vi "Dashboard Main.vi"() -> ()   [LabVIEW 2019]
uses:
  <vilib>/Utility/miscctls.llb/LVRowAndColumnTypeDef.ctl
  <vilib>/event_ctls.llb/eventvkey.ctl
  <vilib>/Rock Robotics/Network Tables/NT Read Numeric Array.vi
  <vilib>/Rock Robotics/WPI/Dashboard/WPI_DashboardLogging Global.vi
  <vilib>/Rock Robotics/Network Tables/NT Write Boolean.vi
panel:
  in  "Camera Settings Right":T1={"Frame Rate"=30, "Compression"=30, "Size"=1, "DB Camera Config"=FALSE} {"Frame Rate" scale=1.0..30.0; "Compression" scale=100.0..-1.0; "Size" items=["640x480", "320x240", "160x120"]}
  in  "Camera Name Right":string(combo)="No Camera Selection"
  out "Camera Perf":string
  in  "Camera Settings":T1={"Frame Rate"=30, "Compression"=30, "Size"=1, "DB Camera Config"=FALSE} {"Frame Rate" scale=1.0..30.0; "Compression" scale=100.0..-1.0; "Size" items=["640x480", "320x240", "160x120"]}
  in  "TCP":refnum<k5>
  in  "Rec Mode":enum32{"Stop", "Record", "Playback"}(radio)
  out "Robot IP":string
  out "Image Message":string="Timeout in Camera Communications"
  in  "Dashboard Tab":T2(tab)
  in  "Enable Vision":bool=TRUE
  out "Vision Enabled":bool=TRUE
  in  "Select Auto":string(combo)="Select Autonomous ..."
  out "NT Connection":bool
  out "MotorChart R":cluster{"Numeric":dbl, "Numeric":dbl}(graph)
  out "MotorChart L":cluster{"Numeric":dbl, "Numeric":dbl}(graph)
  out "MotorSliders R":cluster{"MotorSlide1":dbl, "MotorSlide2":dbl} {"MotorSlide2" scale=-1.0..1.0 scale format="%#_2e"; "MotorSlide1" scale=-1.0..1.0 scale format="%#_2e"}
  out "MotorSliders L":cluster{"MotorSlide1":dbl, "MotorSlide2":dbl} {"MotorSlide2" scale=-1.0..1.0 scale format="%#_2e"; "MotorSlide1" scale=-1.0..1.0 scale format="%#_2e"}
  out "JS1 Z":dbl(slide) scale=-1.0..1.0 scale format="%#_2e"
  out "JS1 Graph":cluster{"X":dbl, "Y":dbl}[](graph)
  out "JS1 Buttons":T3
  out "JS2 Z":dbl(slide) scale=-1.0..1.0 scale format="%#_2e"
  out "JS2 Graph":cluster{"X":dbl, "Y":dbl}[](graph)
  out "JS2 Buttons":T3
  out "Mode":T4(ring)=enum."Auto Disabled"
  out "Right Camera Perf":cluster{"Bandwidth (Mbps)":dbl, "FPS":dbl}
  out "Top RPM":dbl caption="DB/String 1"
  out "Bottom RPM":dbl caption="DB/String 1"
  out "Camera Image Right":T5(plugin-control)
  out "Target Distance":dbl
  out "Skew":dbl caption="DB/String 1"
  out "Area":dbl caption="DB/String 1"
  out "Offset X":dbl
  out "Offset Y":dbl
  in  "Test Slider":dbl(slide) scale=0.0..100.0 scale format="%#_3g"
  in  "On/Off":bool caption="Solenoid"
  in  "Test Name":u16(ring) items=["Select the test to run..."]
  in  "Test Tree":string(tree)
  in  "Motor":cluster{"Value":dbl, "Enable":bool} {"Value" scale=-1.0..1.0 scale format="%#_3g"}
  out "Progress":T6 {"Test Progress" scale=0.0..100.0}
  in  "Rev/Fwd":cluster{"Forward":bool, "Reverse":bool}
  in  "Test Ring":u16(ring) items=["Monochrome", "Color"]
  out "Cmd Status":string
  in  "Execute Command":bool
  in  "Command Params":string[][](table)
  in  "Command Selection":i32(listbox)
  in  "CheckList":i32(listbox)
  out "Tree":string(tree)
  out "Camera Image":T5(plugin-control)
  out "Background":bool
  in  "Camera Name":string(combo)="No Camera Selection"
  # "HW"
  # "HW"
  # "Operator 1"
  # "Operator 2"
  # "Drive Motors"
  # "Front"
  # "Right"
  # "Left"
  # "Back"
  # "This tab is a great place for autonomous settings and robot-specific values.\nPlace controls and indicators inside this tab and match name to\nDashboard Variables on robot. You can also delete this comment."
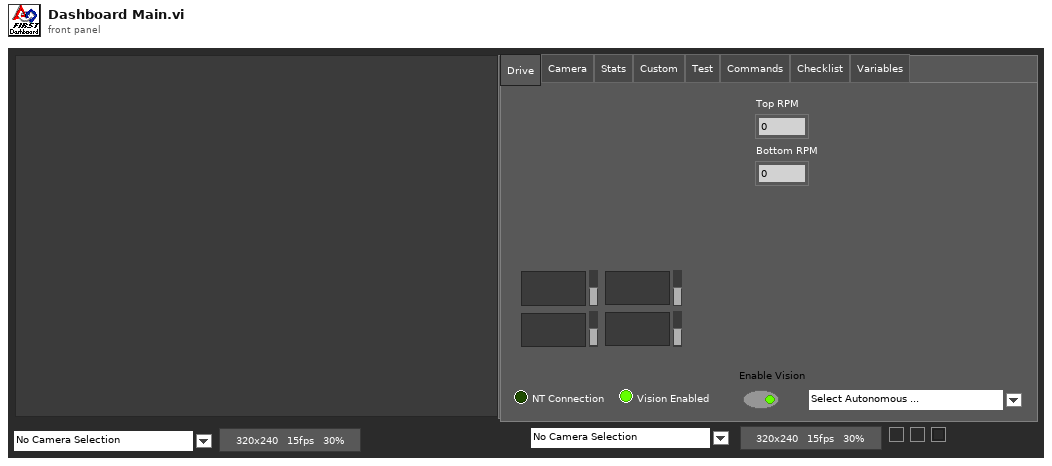
[diagram p1: front panel]
types:
  T1 = cluster{"Frame Rate":i32, "Compression":i32, "Size":u16, "DB Camera Config":bool}
  T2 = enum32{"Drive", "Camera", "Stats", "Custom", "Test", "Commands", "Checklist", "Variables"}
  T3 = cluster{bool, bool, bool, bool, bool, bool, bool, bool, bool, bool, bool, bool}
  T4 = enum8{"Tele-Op Disabled", "Tele-Op Enabled", "Auto Disabled", "Auto Enabled", "Test Disabled", "Test Enabled", "Disconnected", "No Code", "E-Stop"}
  T5 = typedef "IMAQ Image.ctl" = refnum<image>
  T6 = cluster{"Test Progress":u8, "Test Progress Text":string}
  T7 = cluster{"Save Path":path, "Interval (s)":dbl, "Keep":i32}
  T8 = enum32{"Drive", "Camera", "Basic", "Custom", "Test", "Commands", "Checklist", "Variables"}
  T9 = typedef "Image Type" = u32
  T10 = cluster{"IDs":cluster{"RPC field ID":u16, "Unique ID":u16}, "String":string}
  T11 = cluster{"Camera Image":refnum<vi>, "Dashboard Tab":refnum<vi>, "Background":refnum<vi>, "Rec Mode":refnum<vi>, "Test Slider":refnum<vi>, "On/Off ":refnum<vi>, "Test Ring":refnum<vi>, "Rev/Fwd":refnum<vi>, "Test Name":refnum<vi>, "Motor":refnum<vi>, "Progress":refnum<vi>, "CheckList":refnum<vi>, "Tree":refnum<vi>, "Test Tree":refnum<vi>, "Command Params":refnum<vi>, "Command Selection":refnum<vi>, "Execute Command":refnum<vi>, "Cmd Status":refnum<vi>, "Camera Settings":refnum<vi>, "Camera Name":refnum<vi>, "Camera Perf":refnum<vi>, "Camera Settings Right":refnum<vi>, "Camera Name Right":refnum<vi>, "Camera Image Right":refnum<vi>}
  T12 = cluster{"Global Rectangle":i32[], "Contours":cluster{"Contour Type":u32, "ROI Type":u32, "Points":i32[]}[]}
  T13 = cluster{"Camera Name Right":string, string, "Saved DB Images Info":cluster{"Save Path":path, "Interval (s)":dbl, "Keep":i32}}
  T14 = cluster{"Error Strings":string, "Disable Counts":cluster{u16, u16}, "Rail Faults":cluster{u16, u16, u16}, "Robot IP":string, "DB Mode":u8, "Event Info":cluster{"Name":string, "Type":u8, "Number":u16, "Replay":u8}}
  T15 = cluster{"Storage":cluster{"Disk Free":u64, "RAM Block":u32, "RAM free":u32}, "CPU Utilization":cluster{"CPU % ISR":sgl, "CPU % Time Crit":sgl, "CPU % Timed Str":sgl, "CPU % High":sgl, "CPU % Above":sgl, "CPU % Normal":sgl, "CPU % Low":sgl}, "CAN":cluster{"% Bus Utilization":sgl, "Bus Off Cnt":u32, "TX_FIFO Full Cnt":u32, "Receive Error Cnt":u8, "Transmit Error Cnt":u8}, "HID":cluster{"HID Outputs":u32, "Rumble Low":u16, "Rumble High":u16}[]}
  T16 = cluster{"Status bits":cluster{"Test Mode":bool, "Autonomous":bool, "Enabled":bool, "Code Start":bool, "Brownout":bool, "Reserved 2":bool, "Reserved 3":bool, "E-Stop":bool}, "Code Trace":cluster{"Disabled":bool, "TeleOp":bool, "Auto":bool, "Test":bool}, "Controller Type":enum16{"unknown", "cRIO", "roboRio"}, "Code?":enum16{"unknown", "noCode", "code"}, "Battery V":dbl}
  T17 = cluster{"Control Bits":cluster{"TestMode":bool, "Autonomous":bool, "Enabled":bool, "FMS Present":bool, bool, bool, bool, "E-Stop":bool}, "Team Station ":u8, "Countdown":sgl, "Joystick Values":cluster{"Axes":dbl[], "Buttons":bool[], "POVs":i16[]}[]}
  T18 = cluster{"Axes":dbl[], "Buttons":bool[], "POVs":i16[]}[]
  T19 = cluster{"Axes":dbl[], "Buttons":bool[], "POVs":i16[]}
  T20 = cluster{"Buttons[0]":bool, "Buttons[1]":bool, "Buttons[2]":bool, "Buttons[3]":bool, "Buttons[4]":bool, "Buttons[5]":bool, "Buttons[6]":bool, "Buttons[7]":bool, "Buttons[8]":bool, "Buttons[9]":bool, "Buttons[10]":bool, "Buttons[11]":bool}
  T21 = cluster{"Camera Name":string, string, "Saved DB Images Info":cluster{"Save Path":path, "Interval (s)":dbl, "Keep":i32}}
  T22 = cluster{"Operation":enum16{"Update", "Clear"}, "Color Box":u32}[]
  T23 = typedef "eventvkey.ctl" = enum16{"ASCII", "Enter", "Return", "Shift", "Ctrl", "Alt", "Cmd", "Opt", "Caps", "NumLock", "Clear", "Break", "Up", "Down", "Left", "Right", "Insert", "Delete", "Home", "End", "PageUp", "PageDown", "Escape", "Help", "Pause", "ScrollLock", "F1", "F2", "F3", "F4", "F5", "F6", "F7", "F8", "F9", "F10", "F11", "F12", "F13", "F14", "F15", "F16", "F17", "F18", "F19", "F20", "F21", "F22", "F23", "F24", "Play", "VolumeUp", "VolumeDown", "Mute", "Two Byte Char"}
  T24 = cluster{"Image Size":bool, "Image Type":bool, "Pixel Value":bool, "ROI Information":bool, "Zoom Factor":bool}
  T25 = cluster{"Operation":enum16{"Update", "Clear"}, "Color Box":u32}
  T26 = typedef "LVRowAndColumnTypeDef.ctl" = cluster{"Row":i32, "Column":i32}
  T27 = cluster{"Shift":bool, "Ctrl":bool, "Alt":bool, "Cmd":bool, "Opt":bool}
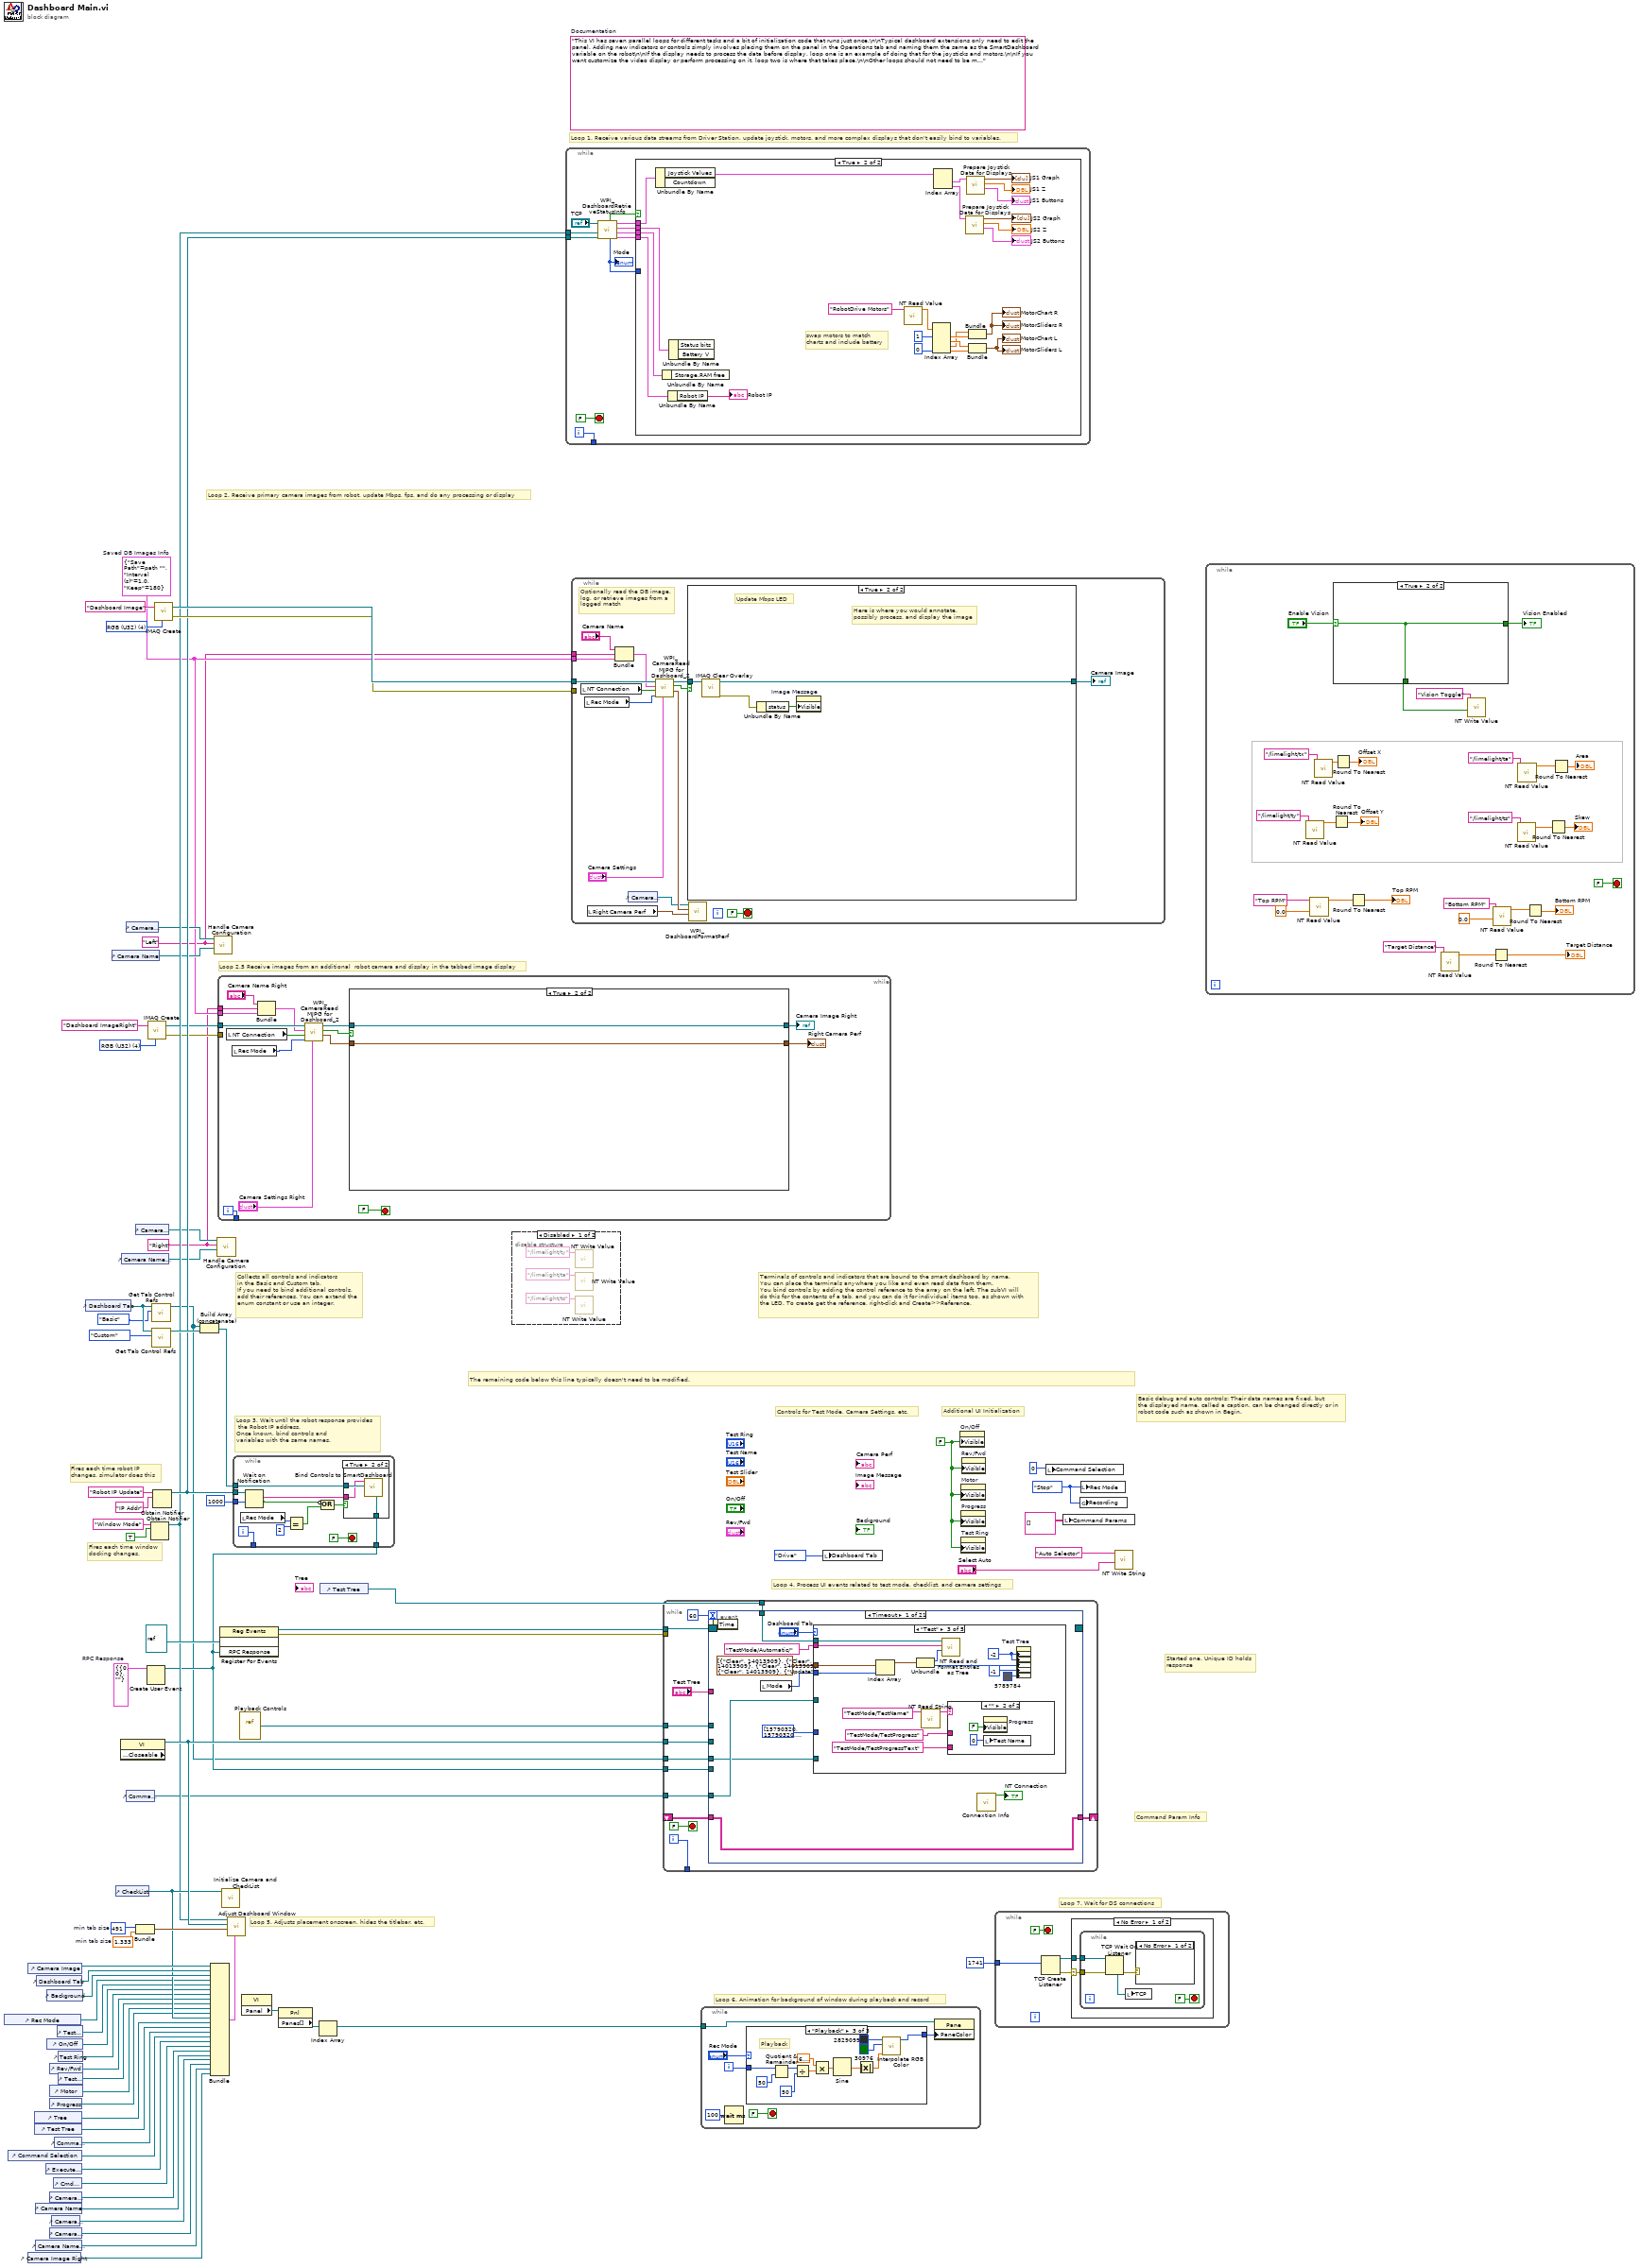
[diagram p0: block diagram]
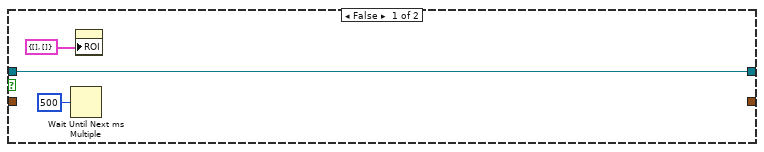
[diagram p4: hidden frame]
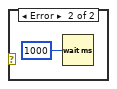
[diagram p5: hidden frame]
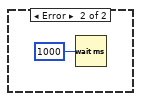
[diagram p6: hidden frame]
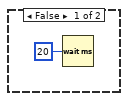
[diagram p7: hidden frame]
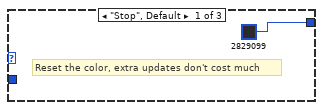
[diagram p8: hidden frame]
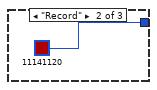
[diagram p9: hidden frame]
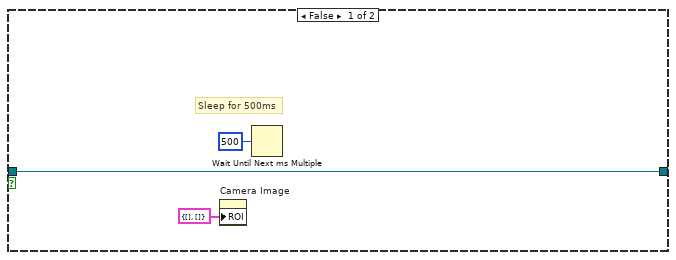
[diagram p11: hidden frame]
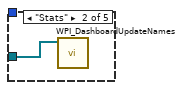
[diagram p13: hidden frame]
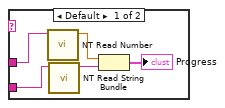
[diagram p14: hidden frame]
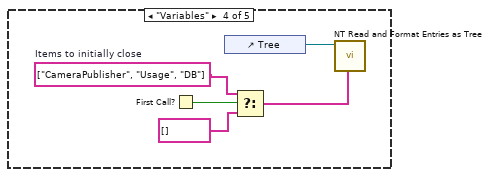
[diagram p15: hidden frame]
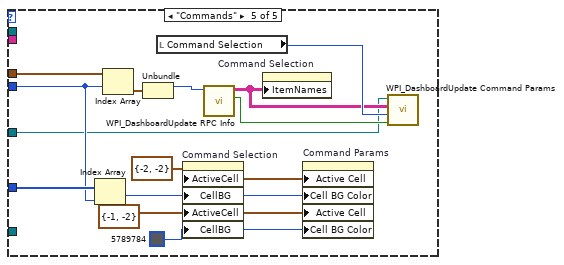
[diagram p16: hidden frame]
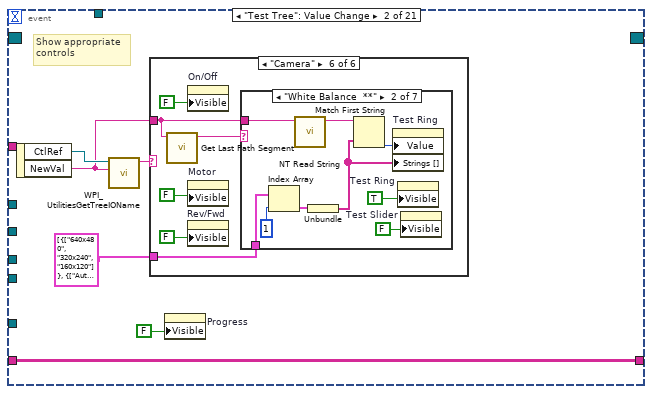
[diagram p17: hidden frame]
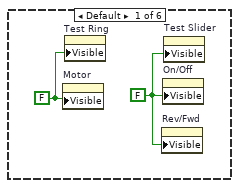
[diagram p18: hidden frame]
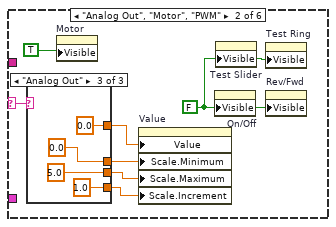
[diagram p19: hidden frame]
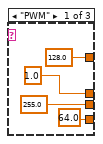
[diagram p20: hidden frame]
diagram:
  w4 = T7 {"Save Path"=path "", "Interval (s)"=1.0, "Keep"=180}  # Saved DB Images Info
  w3 = "Right"
  w2 = "Left"
  w14 = T9 4 items=["Grayscale (U8)", "Grayscale (I16)", "Grayscale (SGL)", "Complex (CSG)", "RGB (U32)", "HSL (U32)", "RGB (U64)"] ("Image Type")
  w30 = T10 {"IDs"={"RPC field ID"=0, "Unique ID"=0}, "String"=""}  # RPC Response
  w52 = 491  # min tab size
  w51 = 1.333  # min tab size
  w59 = enum32{"Stop", "Record", "Playback"}."Stop" ("Rec Mode")
  w36 = FALSE ("Visible")
  (unwired) "This VI has seven parallel loops for different tasks and a bit of initialization code that runs just once.\n\nTypical dashboard extensions only need to edit the panel. Adding new indicators or controls simply involves placing them on the panel in the Operations tab and naming them the same as the SmartDashboard variable on the robot\n\nIf the display needs to process the data before display, loop one is an example of doing that for the joysticks and motors.\n\nIf you want customize the video display or perform processing on it, loop two is where that takes place.\n\nOther loops should not need to be modified. They are pretty standard, and document the task they perform."  # Documentation
  w76 = T9 4 items=["Grayscale (U8)", "Grayscale (I16)", "Grayscale (SGL)", "Complex (CSG)", "RGB (U32)", "HSL (U32)", "RGB (U64)"] ("Image Type")
  # "Loop 2.5 Receive images from an additional  robot camera and display in the tabbed image display"
  # "Command Param Info"
  # "Started one, Unique ID holds\nresponse"
  # "Loop 7. Wait for DS connections"
  # "Basic debug and auto controls: Their data names are fixed, but\nthe displayed name, called a caption, can be changed directly or in\nrobot code such as shown in Begin."
  # "Controls for Test Mode, Camera Settings, etc."
  # "Additional UI Initialization"
  # "Loop 6. Animation for background of window during playback and record"
  # "Fires each time robot IP\nchanges, simulator does this"
  # "Fires each time window\ndocking changes."
  # "Collects all controls and indicators\nin the Basic and Custom tab.\nIf you need to bind additional controls,\nadd their references. You can extend the\nenum constant or use an integer."
  # "The remaining code below this line typically doesn't need to be modified."
  # "Loop 4. Process UI events related to test mode, checklist, and camera settings"
  # "Terminals of controls and indicators that are bound to the smart dashboard by name.\nYou can place the terminals anywhere you like and even read data from them.\nYou bind controls by adding the control reference to the array on the left. The subVI will\ndo this for the contents of a tab, and you can do it for individual items too, as shown with\nthe LED. To create get the reference, right-click and Create>>Reference."
  # "Loop 3. Wait until the robot response provides\n the Robot IP address.\nOnce known, bind controls and\nvariables with the same names."
  # "Loop 5. Adjusts placement onscreen, hides the titlebar, etc."
  # "Loop 1. Receive various data streams from Driver Station, update joystick, motors, and more complex displays that don't easily bind to variables."
  # "Loop 2. Receive primary camera images from robot, update Mbps, fps, and do any processing or display"
  n1 = control-ref of="Rec Mode"() -> (w42:refnum<vi>)
  n2 = control-ref of="Command Selection"() -> (w29:refnum<vi>)
  n3 = control-ref of="Camera Image Right"() -> (w7:refnum<vi>)
  n4 = control-ref of="Camera Image"() -> (w54:refnum<vi>)
  n5 = control-ref of="Tree"() -> (w46:refnum<vi>)
  n6 = control-ref of="Test Tree"() -> (w45:refnum<vi>)
  n7 = control-ref of="Camera Name"() -> (w20:refnum<vi>)
  n8 = control-ref of="Camera Name Right"() -> (w8:refnum<vi>)
  n9 = control-ref of="Dashboard Tab"() -> (w53:refnum<vi>)
  n10 = control-ref of="Execute Command"() -> (w31:refnum<vi>)
  n11 = control-ref of="Background"() -> (w49:refnum<vi>)
  n12 = control-ref of="On/Off"() -> (w40:refnum<vi>)
  n13 = control-ref of="Progress"() -> (w37:refnum<vi>)
  n14 = control-ref of="Camera Settings"() -> (w21:refnum<vi>)
  n15 = control-ref of="Camera Settings Right"() -> (w9:refnum<vi>)
  n16 = control-ref of="Rev/Fwd"() -> (w38:refnum<vi>)
  n17 = control-ref of="Motor"() -> (w43:refnum<vi>)
  n18 = control-ref of="Camera Perf"() -> (w19:refnum<vi>)
  n19 = control-ref of="Cmd Status"() -> (w25:refnum<vi>)
  n20 = control-ref of="Command Params"() -> (w32:refnum<vi>)
  n21 = control-ref of="Test Slider"() -> (w41:refnum<vi>)
  n22 = control-ref of="Test Ring"() -> (w39:refnum<vi>)
  n23 = control-ref of="Test Name"() -> (w44:refnum<vi>)
  n24 = control-ref of="Dashboard Tab"() -> (w57:refnum<vi>)
  n25 = control-ref of="Camera Name"() -> (w22:refnum<vi>)
  n26 = control-ref of="CheckList"() -> (w47:refnum<vi>)
  n27 = property class="VI" props=["Front Panel.Closeable"]() -> (reference out=w58:refnum<vi>)  [unwired: 2 in, 2 out]
  n28 = control-ref of="Camera Name Right"() -> (w10:refnum<vi>)
  n29 = control-ref of="Camera Settings"() -> (w23:refnum<vi>)
  n30 = control-ref of="Command Params"() -> (w24:refnum<vi>)
  n31 = control-ref of="Camera Settings Right"() -> (w11:refnum<vi>)
  n32 = Bundle("min tab size"=w52, "min tab size"=w51) -> (w50:cluster{"min tab size":i32, "min tab size":dbl})  [unwired: 1 in]
  n33 = Create User Event(user event datatype=w30) -> (user event=w26:refnum<user-event>)  [unwired: 1 in, 1 out]
  n34 = call "IMAQ Create"("Image Name"="Dashboard ImageRight", "Image Type"=w14) -> ("New Image"=w13:T5, "error out"=w12:errorcluster)  [unwired: 2 in, 1 out]
  n35 = Obtain Notifier(name (unnamed)="Window Mode", notification data type=TRUE) -> (notifier out=w34:refnum<notifier>)  [unwired: 2 in, 2 out]
  n36 = call <vilib>:"Get Tab Control Refs.vi"("Page Index"=T8."Basic" ("Dashboard Tab"), "TabControl in"=w57) -> ("ControlsOnPage"=w18:refnum<vi>[])  [unwired: 9 in]
  n37 = call <vilib>:"Get Tab Control Refs.vi"("Page Index"=T8."Custom" ("Dashboard Tab"), "TabControl in"=w57) -> ("ControlsOnPage"=w56:refnum<vi>[])  [unwired: 9 in]
  n38 = Obtain Notifier(name (unnamed)="Robot IP Update", notification data type="IP Addr" ("name (unnamed)")) -> (notifier out=w35:refnum<notifier>)  [unwired: 2 in, 2 out]
  n39 = call "IMAQ Create"("Image Name"="Dashboard Image", "Image Type"=w76) -> ("New Image"=w74:T5, "error out"=w73:errorcluster)  [unwired: 2 in, 1 out]
  n40 = Build Array (concatenate)(w18, w56) -> (w55:refnum<vi>[])
  n41 = Bundle("Camera Image"=w54, "Dashboard Tab"=w53, "Background"=w49, "Rec Mode"=w42, "Test Slider"=w41, "On/Off"=w40, "Test Ring"=w39, "Rev/Fwd"=w38, "Test Name"=w44, "Motor"=w43, "Progress"=w37, "CheckList"=w47, "Tree"=w46, "Test Tree"=w45, "Command Params"=w32, "Command Selection"=w29, "Execute Command"=w31, "Cmd Status"=w25, "Camera Settings"=w21, "Camera Name"=w20, "Camera Perf"=w19, "Camera Settings Right"=w9, "Camera Name Right"=w8, "Camera Image Right"=w7) -> (w48:T11)  [unwired: 1 in]
  n42 = call "Handle Camera Configuration.vi"("CameraNameRef"=w22, "Display Name"=w2, "ClusterRef"=w23) -> ()  [unwired: 9 in]
  n43 = call "Handle Camera Configuration.vi"("CameraNameRef"=w10, "Display Name"=w3, "ClusterRef"=w11) -> ()  [unwired: 9 in]
  n44 = while {
    tunnel: w13 -> [w91]
    tunnel: w12 -> [_]
    tunnel: [w86] -> _
    tunnel: w4 -> [w83]
    tunnel: w3 -> [w80]
    i -> [w86]
    stop <- FALSE stop-if-true
    n45 = local read "NT Connection"() -> (w84:bool)
    n46 = local read "Rec Mode"() -> (w90:enum32{"Stop", "Record", "Playback"})
    n47 = Bundle("Camera Name Right"="Camera Name Right", w80, "Saved DB Images Info"=w83) -> (w82:T13)  [unwired: 1 in]
    n48 = call <vilib>:"WPI_CameraRead MJPG for Dashboard_2.vi"("Camera Settings"="Camera Settings Right", "Rec Mode"=w90, "NT Connection"=w84, "Capture Info"=w82, "Image in"=w91) -> ("perf info"=w78:cluster{"Bandwidth (Mbps)":dbl, "fps":dbl}, "Active"=w85:bool, "Image\\ out"=w88:T5)  [unwired: 4 in]
    n49 = case shown="True" w85 {
      tunnel: w88 -> [w93 w95]
      tunnel: [w93 w95] -> w77
      tunnel: [_ w96] -> w79
      tunnel: w78 -> [_ w96]
      frame False {
        n50 = Wait Until Next ms Multiple(millisecond multiple=u32 500) -> ()  [unwired: 1 out]
        n51 = property on="Camera Image Right" class="ImageControl"("ROI"=T12 {"Global Rectangle"=[], "Contours"=[]}) -> ()  [unwired: 2 in, 2 out]
      }
      frame True {
      }
    }
    "Right Camera Perf" <- w79
    "Camera Image Right" <- w77
  }
  n52 = register-events(refnum<vi> refnum, w26) -> (reference out=w63:refnum<event-registration>, error out=w62:errorcluster)  [unwired: 2 in]
  n53 = call "Initialize Camera and CheckList.vi"("ListBox in"=w47) -> ()  [unwired: 11 in]
  n54 = call "Adjust Dashboard Window.vi"("Sizing Refnums"=w48, "Size Constraints"=w50, "VI"=w58, "WIn Mode"=w34) -> ()  [unwired: 8 in]
  n55 = while {
    tunnel: w55 -> [w108]
    tunnel: w35 -> [w106]
    tunnel: [w104] -> _
    tunnel: u32 1000 ("milliseconds to wait") -> [w103]
    tunnel: w26 -> [w97]
    i -> [w104]
    stop <- FALSE stop-if-true
    n56 = local read "Rec Mode"() -> (w99:enum32{"Stop", "Record", "Playback"})
    n57 = Wait on Notification(notifier=w106, timeout in ms (-1)=w103) -> (notification=w105:string, timed out?=w101:bool)  [unwired: 2 in, 2 out]
    n58 = Equal?(x=w99, y=u16 2 ("Rec Mode")) -> (x = y?=w100:bool)
    n59 = Compound Arithmetic op=OR(invert w101, w100) -> (w102:bool)
    n60 = case shown="True" w102 {
      tunnel: w108 -> [_ w111]
      tunnel: w105 -> [_ w110]
      tunnel: w97 -> [_ w109]
      frame False {
      }
      frame True {
        n61 = call <vilib>:"Bind Controls to SmartDashboard.vi"("RPC ref"=w109, "Bound Control Refs"=w111, "Server IP Address"=w110) -> ()  [unwired: 9 in]
      }
    }
  }
  n62 = vi-ref "Playback Controls.vi"() -> (w64:refnum<vi>)
  n63 = property class="VI"() -> ("Panel"=w66:refnum<vi>)  [unwired: 2 in, 2 out]
  n64 = property class="Pnl"(reference=w66) -> ("Panes[]"=w67:refnum<vi>[])  [unwired: 1 in, 2 out]
  n65 = Index Array(array=w67) -> (element=w65:refnum<vi>)  [unwired: 1 in]
  n66 = control-ref of="Test Tree"() -> (w68:refnum<vi>)
  n67 = disable-structure shown="Disabled" {
    frame Disabled {
      n68 = call-poly <vilib>:"NT Write Value.vi"("Name"="/limelight/ty") -> ()  [unwired: 10 in, 1 out]
      n69 = call-poly <vilib>:"NT Write Value.vi"("Name"="/limelight/ta") -> ()  [unwired: 10 in, 1 out]
      n70 = call-poly <vilib>:"NT Write Value.vi"("Name"="/limelight/ts") -> ()  [unwired: 10 in, 1 out]
    }
    frame Enabled {
    }
  }
  n71 = while {
    tunnel: [w124] -> _
    tunnel: w35 -> [w118]
    tunnel: w34 -> [w115]
    i -> [w124]
    stop <- FALSE stop-if-true
    n72 = call <vilib>:"WPI_DashboardRetrieveStatusInfo.vi"("Binding Refnum"=w118, "Window Mode Notifier"=w115, "TCP Cnx"="TCP") -> ("Power and Errors"=w119:T14, "Robot Metrics"=w122:T15, "Status Info"=w123:T16, "Control Info"=w120:T17, "Robot Mode"=w117:T4, "Process?"=w121:bool)  [unwired: 3 in]
    "Mode" <- w117
    n73 = case shown="True" w121 {
      tunnel: w123 -> [_ w150]
      tunnel: w122 -> [_ w149]
      tunnel: w120 -> [_ w148]
      tunnel: w119 -> [_ w147]
      tunnel: w117 -> [_ _]
      frame False {
        n74 = Wait (ms)(milliseconds to wait=u32 20) -> ()  [unwired: 1 out]
      }
      frame True {
        # "swap motors to match\ncharts and include battery"
        n75 = Unbundle By Name(w148) -> ("Joystick Values"=w138:T18)  [unwired: 1 out]
        n76 = Unbundle By Name(w149) -> ()  [unwired: 1 out]
        n77 = Unbundle By Name(w147) -> ("Robot IP"=→"Robot IP":string)
        n78 = Unbundle By Name(w150) -> ()  [unwired: 2 out]
        n79 = call-poly <vilib>:"NT Read Value.vi"("Name"="RobotDrive Motors") -> ("Numeric Array"=w128:dbl[])  [unwired: 9 in, 1 out]
        n80 = Index Array(array=w128, index #1=1, index #4=0) -> (element #1=w142:dbl, element #2=w143:dbl, element #3=w141:dbl, element #4=w146:dbl)  [unwired: 2 in]
        n81 = Index Array(array=w138) -> (element #1=w137:T19, element #2=w133:T19)  [unwired: 2 in]
        n82 = call "Prepare Joystick Data for Displays.vi"("Joystick Values"=w133) -> ("Buttons"=→"JS2 Buttons":T20, "Z Axis"=→"JS2 Z":dbl, "Cartesian Data"=→"JS2 Graph":cluster{"X axis":dbl, "X axis":dbl}[])  [unwired: 8 in]
        n83 = call "Prepare Joystick Data for Displays.vi"("Joystick Values"=w137) -> ("Buttons"=→"JS1 Buttons":T20, "Z Axis"=→"JS1 Z":dbl, "Cartesian Data"=→"JS1 Graph":cluster{"X axis":dbl, "X axis":dbl}[])  [unwired: 8 in]
        n84 = Bundle("Numeric"=w141, "Numeric"=w142) -> (→"MotorChart R" →"MotorSliders R":cluster{"Numeric":dbl, "Numeric":dbl})  [unwired: 1 in]
        n85 = Bundle("Numeric"=w143, "Numeric"=w146) -> (→"MotorChart L" →"MotorSliders L":cluster{"Numeric":dbl, "Numeric":dbl})  [unwired: 1 in]
      }
    }
  }
  n86 = while {
    tunnel: w74 -> [w164]
    tunnel: w73 -> [_]
    tunnel: w4 -> [w158]
    tunnel: w2 -> [w155]
    stop <- FALSE stop-if-true
    # "Optionally read the DB image,\nlog, or retrieve images from a\nlogged match"
    n87 = local read "NT Connection"() -> (w159:bool)
    n88 = local read "Rec Mode"() -> (w161:enum32{"Stop", "Record", "Playback"})
    n89 = local read "Right Camera Perf"() -> (w153:cluster{"Bandwidth (Mbps)":dbl, "FPS":dbl})
    n90 = Bundle("Camera Name"="Camera Name", w155, "Saved DB Images Info"=w158) -> (w157:T21)  [unwired: 1 in]
    n91 = control-ref of="Camera Perf"() -> (w152:refnum<vi>)
    n92 = call <vilib>:"WPI_CameraRead MJPG for Dashboard_2.vi"("Camera Settings"="Camera Settings", "Rec Mode"=w161, "NT Connection"=w159, "Capture Info"=w157, "Image in"=w164) -> ("perf info"=w154:cluster{"Bandwidth (Mbps)":dbl, "fps":dbl}, "Active"=w162:bool, "Image\\ out"=w163:T5)  [unwired: 4 in]
    n93 = case shown="True" w162 {
      tunnel: w163 -> [w167 w170]
      tunnel: [w167 w169] -> w151
      frame False {
        # "Sleep for 500ms"
        n94 = property on="Camera Image" class="ImageControl"("ROI"=T12 {"Global Rectangle"=[], "Contours"=[]}) -> ()  [unwired: 2 in, 2 out]
        n95 = Wait Until Next ms Multiple(millisecond multiple=u32 500) -> ()  [unwired: 1 out]
      }
      frame True {
        # "Here is where you would annotate,\npossibly process, and display the image"
        # "Update Mbps LED"
        n96 = call "IMAQ Clear Overlay"("Image"=w170) -> ("error out"=w171:errorcluster, "Image Out"=w169:T5)  [unwired: 2 in, 7 out]
        n97 = Unbundle By Name(w171) -> ("status"=w172:bool)
        n98 = property on="Image Message" class="Str"("Visible"=w172) -> ()  [unwired: 2 in, 2 out]
      }
    }
    "Camera Image" <- w151
    n99 = call <vilib>:"WPI_DashboardFormatPerf.vi"("Right Camera Perf"=w153, "Performance"=w154, "String in"=w152) -> ()  [unwired: 9 in]
  }
  n100 = while {
    tunnel: [w182] -> _
    tunnel: w68 -> [w181]
    tunnel: w64 -> [w180]
    tunnel: w63 -> [w179]
    tunnel: w62 -> [_]
    tunnel: w58 -> [w178]
    tunnel: w26 -> [w177]
    tunnel: w24 -> [w176]
    shift-right: [w175] -> _
    shift-left: _ -> [w174]
    tunnel: w18 -> [w173]
    i -> [w182]
    stop <- FALSE stop-if-true
    n101 = event shown="[0] Timeout" {
      selector: w179 -> [_ _ _ _ _ _ _ _ _ _ _ _ _ _ _ _ _ _ _ _ _]
      dyn-events: [_ _ _ _ _ _ _ _ _ _ _ _ _ _ _ _ w442 _ _ _ _] -> _
      timeout: u32 60 ("milliseconds to wait") -> [_ _ _ _ _ _ _ _ _ _ _ _ _ _ _ _ _ _ _ _ _]
      tunnel: w181 -> [w194 _ _ _ _ _ _ _ _ _ _ _ _ _ _ _ _ _ _ _ _]
      tunnel: "Test Tree" -> [_ _ _ _ _ _ _ _ _ _ _ w409 w417 w419 w423 w431 _ _ _ _ _]
      tunnel: w180 -> [_ _ _ _ _ _ _ _ _ _ _ _ _ _ _ _ w444 _ w462 _ _]
      tunnel: w178 -> [_ _ _ _ _ _ _ _ _ _ _ _ _ _ _ _ w440 _ _ _ _]
      tunnel: w177 -> [_ _ _ _ _ _ _ _ _ _ _ _ _ _ _ _ w438 _ _ _ _]
      tunnel: w176 -> [w189 _ _ _ _ _ w360 _ _ _ _ _ _ _ _ _ _ _ _ _ _]
      tunnel: [w188 w237 w339 w344 w353 w357 w358 w367 w377 w384 w396 w408 w415 w418 w422 w430 w437 w457 w459 w463 w476] -> w175
      tunnel: w174 -> [w188 w237 w339 w344 w353 w357 w358 _ _ w384 w396 w408 w415 w418 w422 w430 w437 w457 w459 w463 w476]
      tunnel: w173 -> [w186 _ _ _ _ _ _ _ _ _ _ _ _ _ _ _ _ _ _ _ _]
      event Timeout {
        n102 = event-data() -> ()  [unwired: 1 in, 1 out]
        n103 = local read "Mode"() -> (w191:T4)
        n104 = case shown="\"Test\"" "Dashboard Tab" {
          tunnel: w194 -> [_ _ w210 _ _]
          tunnel: "TestMode/Automatic/" ("Name Pattern") -> [_ _ w209 _ _]
          tunnel: T22 [{"Operation"=enum."Clear", "Color Box"=14013909}, {"Operation"=enum."Clear", "Color Box"=14013909}, {"Operation"=enum."Clear", "Color Box"=14013909}, {"Operation"=enum."Clear", "Color Box"=14013909}, {"Operation"=enum."Update", "Color Box"=14013909}, {"Operation"=enum."Update", "Color Box"=16777215}, {"Operation"=enum."Clear", "Color Box"=14013909}, {"Operation"=enum."Clear", "Color Box"=14013909}, {"Operation"=enum."Clear", "Color Box"=14013909}] -> [_ _ w202 _ w230]
          tunnel: w191 -> [_ _ w201 _ w229]
          tunnel: u32[] [15790320, 15790320, 15790320, 15790320, 16777215, 16777215, 15790320, 15790320, 15790320] -> [_ _ _ _ w235]
          tunnel: w189 -> [_ _ _ _ w223]
          tunnel: w186 -> [_ w196 _ _ _]
          frame "Custom", Default {
          }
          frame "Stats" {
            n105 = call <vilib>:"WPI_DashboardUpdateNames.vi"("Controls on Tab"=w196) -> ()  [unwired: 11 in]
          }
          frame "Test" {
            w208 = -2 ("Active Item:Row Number")
            n106 = Index Array(array=w202, index=w201) -> (element=w203:T25)
            n107 = Unbundle(w203) -> ("Operation"=w204:enum16{"Update", "Clear"}, "Color Box"=w205:u32)
            n108 = call <vilib>:"NT Read String.vi"("Name"="TestMode/TestName") -> ("String"=w199:string)  [unwired: 9 in, 1 out]
            n109 = call <vilib>:"NT Read and Format Entries as Tree.vi"("Operation"=w204, "Name Pattern"=w209, "Tree Refnum"=w210) -> ()  [unwired: 7 in, 2 out]
            n110 = case shown="\"\"" w199 {
              tunnel: "TestMode/TestProgress" ("Name") -> [w212 _]
              tunnel: "TestMode/TestProgressText" ("Name") -> [w211 _]
              frame Default {
                n111 = call <vilib>:"NT Read Number.vi"("Name"=w212) -> ("Numeric"=w213:dbl)  [unwired: 9 in, 1 out]
                n112 = call <vilib>:"NT Read String.vi"("Name"=w211) -> ("String"=w214:string)  [unwired: 9 in, 1 out]
                n113 = Bundle("Numeric"=w213, "String"=w214) -> (→"Progress":cluster{"Numeric":dbl, "String":string})  [unwired: 1 in]
              }
              frame "" {
                n114 = property on="Progress" class="Clust (strict)"("Visible"=FALSE) -> ()  [unwired: 2 in, 2 out]
                n115 = local write "Test Name"(u16 0) -> ()
              }
            }
            n116 = property on="Test Tree" class="Tree (strict)"("Active Item Row Number"=w208, "ActiveColNum"=w208, "CellBG"=w205, "Active Item Row Number"=-1 ("Active Item:Row Number"), "CellBG"=u32 5789784 ("Color Box")) -> ()  [unwired: 2 in, 2 out]
          }
          frame "Variables" {
            w220 = string[] ["CameraPublisher", "Usage", "DB"]  # Items to initially close
            n117 = First Call?() -> (First Call?: T/F=w221:bool)
            n118 = control-ref of="Tree"() -> (w222:refnum<vi>)
            n119 = Select(t=w220, s=w221, f=string[] []) -> (s? t:f=w218:string[])
            n120 = call <vilib>:"NT Read and Format Entries as Tree.vi"("Tags to  Close"=w218, "Tree Refnum"=w222) -> ()  [unwired: 8 in, 2 out]
          }
          frame "Commands" {
            w231 = u32 5789784 ("Color Box")
            w232 = T26 {"Row"=-1, "Column"=-2} ("Active Cell:Active Cell")
            w234 = T26 {"Row"=-2, "Column"=-2} ("Active Cell:Active Cell")
            n121 = Index Array(array=w235, index=w229) -> (element=w233:u32)
            n122 = Index Array(array=w230, index=w229) -> (element=w228:T25)
            n123 = Unbundle(w228) -> ("Operation"=w227:enum16{"Update", "Clear"})  [unwired: 1 out]
            n124 = local read "Command Selection"() -> (w226:i32)
            n125 = property on="Command Selection" class="MCListbox (strict)"("ActiveCell"=w234, "CellBG"=w233, "ActiveCell"=w232, "CellBG"=w231) -> ()  [unwired: 2 in, 2 out]
            n126 = call <vilib>:"WPI_DashboardUpdate RPC Info.vi"("Operation"=w227) -> ("update"=w225:bool, "commands"=w224:string[][])  [unwired: 9 in]
            n127 = property on="Command Selection" class="MCListbox (strict)"("ItemNames"=w224) -> ()  [unwired: 2 in, 2 out]
            n128 = property on="Command Params" class="Tbl (strict)"("Active Cell"=w234, "Cell BG Color"=w233, "Active Cell"=w232, "Cell BG Color"=w231) -> ()  [unwired: 2 in, 2 out]
            n129 = call <vilib>:"WPI_DashboardUpdate Command Params.vi"("Update"=w225, "NewVal"=w226, "Commands"=w224, "Param Tbl"=w223) -> ()  [unwired: 7 in, 1 out]
          }
        }
        n130 = call <vilib>:"Connextion Info.vi"() -> ("Connected"=→"NT Connection":bool)  [unwired: 10 in, 1 out]
      }
      event "Test Tree": Value Change {
        # "Show appropriate\ncontrols"
        n131 = event-data() -> ("CtlRef"=w240:refnum<vi>, "NewVal"=w238:string)  [unwired: 1 in]
        n132 = call <vilib>:"WPI_UtilitiesGetTreeIOName.vi"("NewVal"=w238, "TreeControl in"=w240) -> ("I/O Name"=w241:string)  [unwired: 9 in]
        n133 = case shown="\"Camera\"" w241 {
          selector: w241 -> [_ w248 _ w270 w279 _]
          tunnel: w238 -> [_ _ w267 w269 _ w286]
          tunnel: cluster{string[]}[] [{["640x480", "320x240", "160x120"]}, {["Auto", "Fixed indoor", "Fixed outdoor 1", "Fixed outdoor 2", "Fixed fluorescent 1", "Fixed fluorescent 2", "Hold current"]}, {["Auto", "Flicker-free 50 Hz", "Flicker-free 60 Hz", "Hold current"]}, {["None", "Prioritize frame rate", "Prioritize image quality"]}, {["Monochrome", "Color"]}] -> [_ _ _ _ _ w285]
          frame Default {
            w243 = FALSE ("Visible")
            w242 = FALSE ("Visible")
            n134 = property on="Motor" class="Clust (strict)"("Visible"=w242) -> ()  [unwired: 2 in, 2 out]
            n135 = property on="Test Ring" class="Ring (strict)"("Visible"=w242) -> ()  [unwired: 2 in, 2 out]
            n136 = property on="Rev/Fwd" class="Clust (strict)"("Visible"=w243) -> ()  [unwired: 2 in, 2 out]
            n137 = property on="On/Off" class="Bool (strict)"("Visible"=w243) -> ()  [unwired: 2 in, 2 out]
            n138 = property on="Test Slider" class="Slide (strict)"("Visible"=w243) -> ()  [unwired: 2 in, 2 out]
          }
          frame "Analog Out", "Motor", "PWM" {
            w249 = FALSE ("Visible")
            n139 = case shown="\"Analog Out\"" w248 {
              tunnel: [1.0 ("Value") -1.0 ("Value") 0.0 ("Value")] -> w247
              tunnel: [255.0 ("Value") 1.0 ("Value") 5.0 ("Value")] -> w246
              tunnel: [128.0 ("Value") 0.0 ("Value") 0.0 ("Value")] -> w245
              tunnel: [64.0 ("Value") 0.5 ("Value") 1.0 ("Value")] -> w244
              frame "PWM" {
              }
              frame "Motor", Default {
              }
              frame "Analog Out" {
              }
            }
            n140 = property on="Motor" class="Clust (strict)"("Visible"=TRUE) -> ()  [unwired: 2 in, 2 out]
            n141 = property on="Value" class="Slide (strict)"("Value"=w245, "Scale.Minimum"=w247, "Scale.Maximum"=w246, "Scale.Increment"=w244) -> ()  [unwired: 2 in, 2 out]
            n142 = property on="On/Off" class="Bool (strict)"("Visible"=w249) -> ()  [unwired: 2 in, 2 out]
            n143 = property on="Test Slider" class="Slide (strict)"("Visible"=w249) -> ()  [unwired: 2 in, 2 out]
            n144 = property on="Test Ring" class="Ring (strict)"("Visible"=w249) -> ()  [unwired: 2 in, 2 out]
            n145 = property on="Rev/Fwd" class="Clust (strict)"("Visible"=w249) -> ()  [unwired: 2 in, 2 out]
          }
          frame "Servo" {
            w265 = FALSE ("Visible")
            n146 = call <vilib>:"NT Read Number.vi"("Name"=w267) -> ("Numeric"=w266:dbl)  [unwired: 9 in, 1 out]
            n147 = property on="Test Slider" class="Slide (strict)"("Visible"=TRUE, "Scale.Maximum"=170.0 ("Scale.Range:Maximum")) -> ()  [unwired: 2 in, 2 out]
            n148 = local write "Test Slider"(w266) -> ()
            n149 = property on="Motor" class="Clust (strict)"("Visible"=w265) -> ()  [unwired: 2 in, 2 out]
            n150 = property on="Rev/Fwd" class="Clust (strict)"("Visible"=w265) -> ()  [unwired: 2 in, 2 out]
            n151 = property on="On/Off" class="Bool (strict)"("Visible"=w265) -> ()  [unwired: 2 in, 2 out]
            n152 = property on="Test Ring" class="Ring (strict)"("Visible"=w265) -> ()  [unwired: 2 in, 2 out]
          }
          frame "Relay", "Solenoid" {
            w268 = FALSE ("Visible")
            n153 = property on="Motor" class="Clust (strict)"("Visible"=w268) -> ()  [unwired: 2 in, 2 out]
            n154 = property on="Test Slider" class="Slide (strict)"("Visible"=w268) -> ()  [unwired: 2 in, 2 out]
            n155 = Search and Replace String(input string=w269, search string="/Value  **", replace string="/Direction") -> (result string=w275:string)  [unwired: 5 in, 3 out]
            n156 = property on="Test Ring" class="Ring (strict)"("Visible"=w268) -> ()  [unwired: 2 in, 2 out]
            n157 = call <vilib>:"NT Read String.vi"("Name"=w275) -> ("String"=w273:string)  [unwired: 9 in, 1 out]
            n158 = Equal?(x="Both directions", y=w273) -> (x = y?=w271:bool)
            n159 = Not(x=w271) -> (.not. x?=w272:bool)
            n160 = property on="Rev/Fwd" class="Clust (strict)"("Visible"=w271) -> ()  [unwired: 2 in, 2 out]
            n161 = property on="On/Off" class="Bool (strict)"("Visible"=w272, "Caption.Text"=w270) -> ()  [unwired: 2 in, 2 out]
          }
          frame "Compressor", "Digital Out" {
            w278 = FALSE ("Visible")
            # "Get direction and finish"
            n162 = property on="Motor" class="Clust (strict)"("Visible"=w278) -> ()  [unwired: 2 in, 2 out]
            n163 = property on="Test Slider" class="Slide (strict)"("Visible"=w278) -> ()  [unwired: 2 in, 2 out]
            n164 = property on="Test Ring" class="Ring (strict)"("Visible"=w278) -> ()  [unwired: 2 in, 2 out]
            n165 = property on="On/Off" class="Bool (strict)"("Visible"=TRUE, "Caption.Text"=w279) -> ()  [unwired: 2 in, 2 out]
            n166 = property on="Rev/Fwd" class="Clust (strict)"("Visible"=FALSE) -> ()  [unwired: 2 in, 2 out]
          }
          frame "Camera" {
            n167 = call <vilib>:"Get Last Path Segment.vi"("String in"=w286) -> ("String out"=w287:string)  [unwired: 10 in]
            n168 = property on="On/Off" class="Bool (strict)"("Visible"=FALSE) -> ()  [unwired: 2 in, 2 out]
            n169 = property on="Motor" class="Clust (strict)"("Visible"=FALSE) -> ()  [unwired: 2 in, 2 out]
            n170 = property on="Rev/Fwd" class="Clust (strict)"("Visible"=FALSE) -> ()  [unwired: 2 in, 2 out]
            n171 = case shown="\"White Balance  **\"" w287 {
              tunnel: w286 -> [w293 w302 w311 w320 w329 _ w335]
              tunnel: w285 -> [w291 w299 w308 w317 w326 _ _]
              frame "Size  **" {
                n172 = Index Array(array=w291) -> (element=w290:cluster{string[]})  [unwired: 1 in]
                n173 = call <vilib>:"NT Read String.vi"("Name"=w293) -> ("String"=w292:string)  [unwired: 9 in, 1 out]
                n174 = Unbundle(w290) -> (w288:string[])
                n175 = Match First String(2:w288, 3:w292) -> (0:w289:i32)  [unwired: 1 out]
                n176 = property on="Test Ring" class="Ring (strict)"("Value"=w289, "Strings []"=w288) -> ()  [unwired: 2 in, 2 out]
                n177 = property on="Test Ring" class="Ring (strict)"("Visible"=TRUE) -> ()  [unwired: 2 in, 2 out]
                n178 = property on="Test Slider" class="Slide (strict)"("Visible"=FALSE) -> ()  [unwired: 2 in, 2 out]
              }
              frame "White Balance  **" {
                n179 = Index Array(array=w299, index=1) -> (element=w300:cluster{string[]})
                n180 = call <vilib>:"NT Read String.vi"("Name"=w302) -> ("String"=w301:string)  [unwired: 9 in, 1 out]
                n181 = Unbundle(w300) -> (w297:string[])
                n182 = Match First String(2:w297, 3:w301) -> (0:w296:i32)  [unwired: 1 out]
                n183 = property on="Test Ring" class="Ring (strict)"("Value"=w296, "Strings []"=w297) -> ()  [unwired: 2 in, 2 out]
                n184 = property on="Test Ring" class="Ring (strict)"("Visible"=TRUE) -> ()  [unwired: 2 in, 2 out]
                n185 = property on="Test Slider" class="Slide (strict)"("Visible"=FALSE) -> ()  [unwired: 2 in, 2 out]
              }
              frame "Exposure  **" {
                n186 = Index Array(array=w308, index=2) -> (element=w309:cluster{string[]})
                n187 = call <vilib>:"NT Read String.vi"("Name"=w311) -> ("String"=w310:string)  [unwired: 9 in, 1 out]
                n188 = Unbundle(w309) -> (w305:string[])
                n189 = Match First String(2:w305, 3:w310) -> (0:w306:i32)  [unwired: 1 out]
                n190 = property on="Test Ring" class="Ring (strict)"("Value"=w306, "Strings []"=w305) -> ()  [unwired: 2 in, 2 out]
                n191 = property on="Test Ring" class="Ring (strict)"("Visible"=TRUE) -> ()  [unwired: 2 in, 2 out]
                n192 = property on="Test Slider" class="Slide (strict)"("Visible"=FALSE) -> ()  [unwired: 2 in, 2 out]
              }
              frame "Exposure Priority  **" {
                n193 = Index Array(array=w317, index=3) -> (element=w318:cluster{string[]})
                n194 = call <vilib>:"NT Read String.vi"("Name"=w320) -> ("String"=w319:string)  [unwired: 9 in, 1 out]
                n195 = Unbundle(w318) -> (w314:string[])
                n196 = Match First String(2:w314, 3:w319) -> (0:w315:i32)  [unwired: 1 out]
                n197 = property on="Test Ring" class="Ring (strict)"("Value"=w315, "Strings []"=w314) -> ()  [unwired: 2 in, 2 out]
                n198 = property on="Test Ring" class="Ring (strict)"("Visible"=TRUE) -> ()  [unwired: 2 in, 2 out]
                n199 = property on="Test Slider" class="Slide (strict)"("Visible"=FALSE) -> ()  [unwired: 2 in, 2 out]
              }
              frame "Color Enable  **" {
                n200 = Index Array(array=w326, index=4) -> (element=w327:cluster{string[]})
                n201 = call <vilib>:"NT Read String.vi"("Name"=w329) -> ("String"=w328:string)  [unwired: 9 in, 1 out]
                n202 = Unbundle(w327) -> (w323:string[])
                n203 = Match First String(2:w323, 3:w328) -> (0:w324:i32)  [unwired: 1 out]
                n204 = property on="Test Ring" class="Ring (strict)"("Value"=w324, "Strings []"=w323) -> ()  [unwired: 2 in, 2 out]
                n205 = property on="Test Ring" class="Ring (strict)"("Visible"=TRUE) -> ()  [unwired: 2 in, 2 out]
                n206 = property on="Test Slider" class="Slide (strict)"("Visible"=FALSE) -> ()  [unwired: 2 in, 2 out]
              }
              frame Default {
                n207 = property on="Test Ring" class="Ring (strict)"("Visible"=FALSE) -> ()  [unwired: 2 in, 2 out]
                n208 = property on="Test Slider" class="Slide (strict)"("Visible"=FALSE) -> ()  [unwired: 2 in, 2 out]
              }
              frame "Brightness  **", "Color Level  **", "Compression  **", "FPS  **", "Sharpness  **" {
                n209 = call <vilib>:"NT Read Number.vi"("Name"=w335) -> ("Numeric"=w334:dbl)  [unwired: 9 in, 1 out]
                n210 = local write "Test Slider"(w334) -> ()
                n211 = property on="Test Slider" class="Slide (strict)"("Visible"=TRUE, "Scale.Maximum"=100.0 ("Scale.Range:Maximum")) -> ()  [unwired: 2 in, 2 out]
                n212 = property on="Test Ring" class="Ring (strict)"("Visible"=FALSE) -> ()  [unwired: 2 in, 2 out]
              }
            }
          }
        }
        n213 = property on="Progress" class="Clust (strict)"("Visible"=FALSE) -> ()  [unwired: 2 in, 2 out]
      }
      event "Test Name": Mouse Enter {
        # "Populate the ring with the list of tests"
        n214 = event-data() -> ()  [unwired: 1 in, 1 out]
        n215 = call <vilib>:"NT Read String Array.vi"("Name"="TestMode/TestList") -> ("String Array"=w343:string[])  [unwired: 9 in, 1 out]
        n216 = Build Array (concatenate)("Select the test to run...", w343) -> (w342:string[])
        n217 = property on="Test Name" class="Ring (strict)"("Strings []"=w342) -> ()  [unwired: 2 in, 2 out]
      }
      event "Test Name": Value Change {
        w345 = FALSE ("Visible")
        # "Tell the robot the test name to run"
        n218 = event-data() -> ("NewVal"=w349:u16)  [unwired: 1 in]
        n219 = property on="Test Name" class="Ring (strict)"() -> ("Strings []"=w350:string[])  [unwired: 2 in, 2 out]
        n220 = local write "Progress"(T6 {"Test Progress"=0, "Test Progress Text"=""} ("Progress")) -> ()
        n221 = Index Array(array=w350, index=w349) -> (element=w348:string)
        n222 = call <vilib>:"NT Write String.vi"("String"=w348, "Name"="TestMode/TestName") -> ()  [unwired: 9 in, 1 out]
        n223 = property on="Progress" class="Clust (strict)"("Visible"=TRUE) -> ()  [unwired: 2 in, 2 out]
        n224 = property on="Motor" class="Clust (strict)"("Visible"=w345) -> ()  [unwired: 2 in, 2 out]
        n225 = property on="Test Slider" class="Slide (strict)"("Visible"=w345) -> ()  [unwired: 2 in, 2 out]
        n226 = property on="On/Off" class="Bool (strict)"("Visible"=w345) -> ()  [unwired: 2 in, 2 out]
        n227 = property on="Rev/Fwd" class="Clust (strict)"("Visible"=w345) -> ()  [unwired: 2 in, 2 out]
        n228 = property on="Test Ring" class="Ring (strict)"("Visible"=w345) -> ()  [unwired: 2 in, 2 out]
      }
      event "Select Auto": Mouse Enter {
        # "Populate the combo box with the list of autonomous options"
        n229 = event-data() -> ()  [unwired: 1 in, 1 out]
        n230 = call <vilib>:"NT Read String Array.vi"("Name"="Auto List") -> ("String Array"=w352:string[])  [unwired: 9 in, 1 out]
        n231 = property on="Select Auto" class="CmbBox"("Strings[]"=w352) -> ()  [unwired: 2 in, 2 out]
      }
      event "Select Auto": Value Change {
        # "User modified the Auto Selection. Write to NT variable so robot knows."
        n232 = event-data() -> ("NewVal"=w355:string)  [unwired: 1 in]
        n233 = call <vilib>:"NT Write String.vi"("String"=w355, "Name"="Auto Selector") -> ()  [unwired: 9 in, 1 out]
      }
      event "Command Selection": Value Change {
        # "Get the params and show in table"
        n234 = event-data() -> ("NewVal"=w361:i32)  [unwired: 1 in]
        n235 = property on="Command Selection" class="MCListbox (strict)"() -> ("ItemNames"=w359:string[][])  [unwired: 2 in, 2 out]
        n236 = call <vilib>:"WPI_DashboardUpdate Command Params.vi"("NewVal"=w361, "Commands"=w359, "Param Tbl"=w360) -> ()  [unwired: 8 in, 1 out]
      }
      event "Execute Command": Value Change {
        # "Started one, Unique ID holds\nresponse"
        n237 = event-data() -> ()  [unwired: 1 in, 1 out]
        n238 = property on="Command Selection" class="MCListbox (strict)"() -> ("ItemNames"=w372:string[][])  [unwired: 2 in, 2 out]
        n239 = Index Array(array=w372, index (row)="Command Selection", index (col)=0) -> (element=w370:string)
        n240 = call <vilib>:"Invoke Commands.vi"("Command Params"="Command Params", "Function Name"=w370) -> ("Params"=w366:u8, "Started"=w365:bool)  [unwired: 7 in, 1 out]
        n241 = Array Subset(array="Command Params", length (row)=w366) -> (w367:string[][])  [unwired: 3 in]
        n242 = Select(t="Executing" ("Cmd Status"), s=w365, f="" ("Cmd Status")) -> (s? t:f=→"Cmd Status":string)
      }
      event "Command Selection": Double Click {
        n243 = event-data() -> ("Row"=w380:i32)  [unwired: 1 in]
        n244 = property on="Command Selection" class="MCListbox (strict)"() -> ("ItemNames"=w383:string[][])  [unwired: 2 in, 2 out]
        n245 = local read "Command Params"() -> (w379:string[][])
        n246 = Index Array(array=w383, index (row)=w380, index (col)=0) -> (element=w381:string)
        n247 = call <vilib>:"Invoke Commands.vi"("Command Params"=w379, "Function Name"=w381) -> ("Params"=w378:u8, "Started"=w373:bool)  [unwired: 7 in, 1 out]
        n248 = Array Subset(array=w379, length (row)=w378) -> (w377:string[][])  [unwired: 3 in]
        n249 = Select(t="Executing" ("Cmd Status"), s=w373, f="" ("Cmd Status")) -> (s? t:f=w374:string)
        n250 = local write "Cmd Status"(w374) -> ()
      }
      event "CheckList": Double Click {
        # "Shift clears all"
        # "Update symbols on the listbox"
        n251 = event-data() -> ("PlatMods.Shift"=w385:bool, "Row"=w387:i32)  [unwired: 1 in]
        n252 = case shown="True" w385 {
          tunnel: w387 -> [w391 _]
          tunnel: 1 -> [w390 _]
          frame False {
            n253 = property on="CheckList" class="LstBox (strict)"() -> ("Item Symbols"=w389:i32[])  [unwired: 2 in, 2 out]
            n254 = Replace Array Subset(array=w389, new element=w390, index=w391) -> (w388:i32[])
            n255 = property on="CheckList" class="LstBox (strict)"("Item Symbols"=w388) -> ()  [unwired: 2 in, 2 out]
          }
          frame True {
            w392 = 0 ("Top Row")
            n256 = property on="CheckList" class="LstBox (strict)"() -> ("Number of Rows"=w394:u32)  [unwired: 2 in, 2 out]
            n257 = Initialize Array(0, w394) -> (w393:i32[])
            n258 = property on="CheckList" class="LstBox (strict)"("Top Row"=w392, "Value"=w392, "Item Symbols"=w393) -> ()  [unwired: 2 in, 2 out]
          }
        }
      }
      event "CheckList": Key Down {
        # "Update symbols on the listbox\nLeft and right keys check and uncheck"
        n259 = event-data() -> ("VKey"=w398:T23)  [unwired: 1 in]
        n260 = case shown="\"Left\", \"Right\"" w398 {
          selector: w398 -> [w403 _]
          tunnel: eventvkey."Left" ("VKey") -> [w401 _]
          frame "Left", "Right" {
            n261 = Equal?(x=w401, y=w403) -> (x = y?=w402:bool)
            n262 = Select(t=0, s=w402, f=1) -> (s? t:f=w404:i32)
            n263 = property on="CheckList" class="LstBox (strict)"() -> ("Item Symbols"=w407:i32[])  [unwired: 2 in, 2 out]
            n264 = Replace Array Subset(array=w407, new element=w404, index="CheckList") -> (w406:i32[])
            n265 = property on="CheckList" class="LstBox (strict)"("Item Symbols"=w406) -> ()  [unwired: 2 in, 2 out]
          }
          frame Default {
          }
        }
      }
      event "Motor.Enable": Value Change {
        # "When the test mode otor enable helper is set, update that\ntree row item's value"
        n266 = event-data() -> ("NewVal"=w413:bool)  [unwired: 1 in]
        n267 = Unbundle("Motor") -> ("Value"=w412:dbl)  [unwired: 1 out]
        n268 = Select(t=w412, s=w413, f=0.0) -> (s? t:f=w410:dbl)
        n269 = call <vilib>:"NT Write Number.vi"("Numeric"=w410, "Name"=w409) -> ()  [unwired: 9 in, 1 out]
      }
      event "Test Slider": Value Change {
        # "When the test mode slider helper is set, update that\ntree row item's value"
        n270 = event-data() -> ("NewVal"=w416:dbl)  [unwired: 1 in]
        n271 = call <vilib>:"NT Write Number.vi"("Numeric"=w416, "Name"=w417) -> ()  [unwired: 9 in, 1 out]
      }
      event "On/Off": Value Change {
        # "When the test mode on/off helper value is set, update that\ntree row item's value"
        n272 = event-data() -> ("NewVal"=w421:bool)  [unwired: 1 in]
        n273 = Boolean To (0,1)(Boolean=w421) -> (0, 1=w420:i16)
        n274 = call <vilib>:"NT Write Number.vi"("Numeric"=w420, "Name"=w419) -> ()  [unwired: 9 in, 1 out]
      }
      event "Rev/Fwd": Value Change {
        # "When the test mode helper value for relays is set, update that\ntree row item's value"
        n275 = event-data() -> ("NewVal.Forward"=w429:bool, "NewVal.Reverse"=w428:bool)  [unwired: 1 in]
        n276 = Boolean To (0,1)(Boolean=w429) -> (0, 1=w425:i16)
        n277 = Boolean To (0,1)(Boolean=w428) -> (0, 1=w427:i16)
        n278 = Negate(x=w427) -> (-x=w426:i16)
        n279 = Add(x=w425, y=w426) -> (x+y=w424:i16)
        n280 = call <vilib>:"NT Write Number.vi"("Numeric"=w424, "Name"=w423) -> ()  [unwired: 9 in, 1 out]
      }
      event "Test Ring": Value Change {
        # "When a test mode helper value is selected from the ring,\nset the tree item's variable to the string value"
        n281 = event-data() -> ("NewVal"=w433:u16)  [unwired: 1 in]
        n282 = property on="Test Ring" class="Ring (strict)"() -> ("Strings []"=w434:string[])  [unwired: 2 in, 2 out]
        n283 = Index Array(array=w434, index=w433) -> (element=w432:string)
        n284 = call <vilib>:"NT Write String.vi"("String"=w432, "Name"=w431) -> ()  [unwired: 9 in, 1 out]
      }
      event "Rec Mode": Value Change {
        # "Update globals for recording mode and path to read log from.\nClear when logging and let NetworkTables set path for vision to\nuse."
        n285 = event-data() -> ("NewVal"=w445:enum32{"Stop", "Record", "Playback"})  [unwired: 1 in]
        n286 = global write "WPI_DashboardLogging Global.vi" "Logging Filename"(path "") -> ()
        n287 = global write "WPI_DashboardLogging Global.vi" "Recording"(w445) -> ()
        n288 = case shown="\"Playback\"" w445 {
          tunnel: w444 -> [_ w447 w456]
          tunnel: [_ _ w455] -> w442
          tunnel: [_ _ w454] -> _
          tunnel: w440 -> [_ _ w452]
          tunnel: cluster{i32, i32} {-250, 170} -> [_ _ w451]
          tunnel: [_ _ T24 {"Image Size"=TRUE, "Image Type"=TRUE, "Pixel Value"=TRUE, "ROI Information"=TRUE, "Zoom Factor"=FALSE} ("Image Information Shown:All Elements")] -> w435
          tunnel: [_ _ TRUE ("Zoom Factor")] -> w436
          tunnel: w438 -> [_ _ w448]
          frame Default {
          }
          frame "Stop", "Record" {
            # "Place Window too"
            n289 = invoke class="VI" method="FP.Close"(reference=w447) -> (reference out=w446:refnum<vi>)  [unwired: 2 in, 2 out]
            n290 = invoke class="VI" method="Abort VI"(reference=w446) -> ()  [unwired: 2 in, 3 out]
          }
          frame "Playback" {
            n291 = call "Open Playback Panel.vi"("Offset"=w451, "DB VI Ref"=w452, "Playback in"=w456) -> ("Playback out"=w453:refnum<vi>)  [unwired: 8 in]
            n292 = register-events(w453, w448) -> (reference out=w455:refnum<event-registration>, error out=w454:errorcluster)  [unwired: 2 in]
          }
        }
        n293 = property on="Camera Image Right" class="ImageControl"("Image Information Shown"=w435, "Image Information Visible"=w436) -> ()  [unwired: 2 in, 2 out]
        n294 = property on="Camera Image" class="ImageControl"("Image Information Shown"=w435, "Image Information Visible"=w436) -> ()  [unwired: 2 in, 2 out]
        n295 = call <vilib>:"WPI_DashboardNT Log FieldName Cache.vi"("Operation"=enum16{"Lookup/Add", "Index", "Clear"}."Clear") -> ()  [unwired: 8 in, 3 out]
      }
      event Panel Close {
        w458 = enum32{"Stop", "Record", "Playback"}."Stop" ("Rec Mode")
        # "Playback window has been closed, abort"
        n296 = event-data() -> ()  [unwired: 1 in, 4 out]
        n297 = local write "Rec Mode"(w458) -> ()
        n298 = global write "WPI_DashboardLogging Global.vi" "Recording"(w458) -> ()
      }
      event Panel Close {
        # "Abort playback window and ourself"
        n299 = event-data() -> ()  [unwired: 1 in, 4 out]
        n300 = invoke class="VI" method="FP.Close"(reference=w462) -> (reference out=w461:refnum<vi>)  [unwired: 2 in, 2 out]
        n301 = invoke class="VI" method="Abort VI"(reference=w461) -> (error out=w460:errorcluster)  [unwired: 2 in, 2 out]
        n302 = invoke class="VI" method="Abort VI"(error in=w460) -> ()  [unwired: 2 in, 3 out]
      }
      event User Event {
        n303 = event-data() -> ("IDs"=w469:cluster{"RPC field ID":u16, "Unique ID":u16}, "String"=w468:string)  [unwired: 1 in]
        n304 = Bundle("IDs"=w469, "String"=w468) -> (w467:T10)  [unwired: 1 in]
        n305 = call <vilib>:"Retrieve RPC Response.vi"("RPC Response"=w467) -> ("Output"=w465:string[][])  [unwired: 10 in]
        n306 = Build Array (concatenate)(w463, w465) -> (w464:string[][])
        n307 = local write "Command Params"(w464) -> ()
        n308 = local write "Cmd Status"("" ("Cmd Status")) -> ()
      }
      event "Tree": Double Click {
        n309 = event-data() -> ("PlatMods"=w475:T27, "Tag"=w472:string)  [unwired: 1 in]
        n310 = Unbundle(w475) -> ("Shift"=w474:bool)  [unwired: 4 out]
        n311 = String Subset(string=w472, length (rest)=1 ("length (rest)")) -> (substring=w471:string)  [unwired: 1 in]
        n312 = Not(x=w474) -> (.not. x?=w473:bool)
        n313 = case shown="\"/\"" w471 {
          tunnel: w472 -> [_ w478]
          tunnel: w473 -> [_ w477]
          frame Default {
          }
          frame "/" {
            n314 = call <vilib>:"NT Update Persistence.vi"("Persistence"=w477, "Name"=w478) -> ()  [unwired: 9 in, 1 out]
          }
        }
      }
    }
  }
  n315 = while {
    tunnel: w65 -> [w480]
    i -> [w483]
    stop <- FALSE stop-if-true
    n316 = Wait (ms)(milliseconds to wait=u32 100) -> ()  [unwired: 1 out]
    n317 = case shown="\"Playback\"" "Rec Mode" {
      tunnel: w483 -> [_ _ w498]
      tunnel: [u32 2829099 ("Base Color") u32 11141120 ("Target Color") w487] -> w479
      frame "Stop", Default {
        # "Reset the color, extra updates don't cost much"
      }
      frame "Record" {
      }
      frame "Playback" {
        # "Playback"
        n318 = Quotient & Remainder(x=w498, y=u32 50 ("milliseconds to wait")) -> (x-y*floor(x/y)=w494:u32)  [unwired: 1 out]
        n319 = Divide(x=w494, y=u32 50 ("milliseconds to wait")) -> (x/y=w491:dbl)
        n320 = Multiply(x=6.283185307179586, y=w491) -> (x*y=w496:dbl)
        n321 = Sine(x=w496) -> (sin(x)=w495:dbl)
        n322 = Absolute Value(x=w495) -> (abs(x)=w488:dbl)
        n323 = call "Interpolate RGB Color.vi"("Proportion"=w488, "Target Color"=u32 30976, "Base Color"=u32 2829099) -> ("Result Color"=w487:u32)  [unwired: 8 in]
      }
    }
    n324 = property class="Pane"(reference=w480, "PaneColor"=w479) -> ()  [unwired: 1 in, 2 out]
  }
  n325 = local write "Dashboard Tab"(T2."Drive" ("Dashboard Tab")) -> ()
  n326 = property on="On/Off" class="Bool (strict)"("Visible"=w36) -> ()  [unwired: 2 in, 2 out]
  n327 = property on="Motor" class="Clust (strict)"("Visible"=w36) -> ()  [unwired: 2 in, 2 out]
  n328 = property on="Progress" class="Clust (strict)"("Visible"=w36) -> ()  [unwired: 2 in, 2 out]
  n329 = property on="Test Ring" class="Ring (strict)"("Visible"=w36) -> ()  [unwired: 2 in, 2 out]
  n330 = property on="Rev/Fwd" class="Clust (strict)"("Visible"=w36) -> ()  [unwired: 2 in, 2 out]
  n331 = while {
    tunnel: u16 1741 ("timeout ms (25000)") -> [w500]
    stop <- FALSE stop-if-true
    n332 = TCP Create Listener(10:w500) -> (0:w499:errorcluster, 3:w501:refnum<k5>)  [unwired: 4 in, 1 out]
    n333 = case shown="No Error" w499 {
      selector: w499 -> [w503 _]
      tunnel: w501 -> [w504 _]
      frame No Error {
        n334 = while {
          tunnel: w504 -> [w507]
          tunnel: w503 -> [w506]
          stop <- FALSE stop-if-true
          n335 = TCP Wait On Listener(8:w506, 11:w507) -> (0:w508:errorcluster, 4:w509:refnum<k5>)  [unwired: 2 in, 3 out]
          n336 = local write "TCP"(w509) -> ()
          n337 = case shown="No Error" w508 {
            frame No Error {
            }
            frame Error {
              n338 = Wait (ms)(milliseconds to wait=u32 1000) -> ()  [unwired: 1 out]
            }
          }
        }
      }
      frame Error {
        n339 = Wait (ms)(milliseconds to wait=u32 1000) -> ()  [unwired: 1 out]
      }
    }
  }
  n340 = local write "Command Selection"(u16 0 ("milliseconds to wait")) -> ()
  n341 = local write "Command Params"(string[][] [] ("Command Params")) -> ()
  n342 = global write "WPI_DashboardLogging Global.vi" "Recording"(w59) -> ()
  n343 = local write "Rec Mode"(w59) -> ()
  n344 = call <vilib>:"NT Write String.vi"("String"="Select Auto", "Name"="Auto Selector") -> ()  [unwired: 9 in, 1 out]
  n345 = while {
    stop <- FALSE stop-if-true
    n346 = call-poly <vilib>:"NT Read Value.vi"("Name"="/limelight/ty") -> ("Numeric"=w517:dbl)  [unwired: 9 in, 1 out]
    n347 = call-poly <vilib>:"NT Read Value.vi"("Default Value"=0.0, "Name"="Top RPM") -> ("Numeric"=w525:dbl)  [unwired: 8 in, 1 out]
    n348 = call-poly <vilib>:"NT Read Value.vi"("Name"="/limelight/tx") -> ("Numeric"=w519:dbl)  [unwired: 9 in, 1 out]
    n349 = Round To Nearest(number=w517) -> (nearest integer value=→"Offset Y":dbl)
    n350 = case shown="True" "Enable Vision" {
      selector: "Enable Vision" -> [w540 w541]
      tunnel: [w540 w541] -> w533
      tunnel: [w540 w541] -> w532
      frame False {
      }
      frame True {
      }
    }
    "Vision Enabled" <- w533
    n351 = Round To Nearest(number=w519) -> (nearest integer value=→"Offset X":dbl)
    n352 = Round To Nearest(number=w525) -> (nearest integer value=→"Top RPM":dbl)
    n353 = call-poly <vilib>:"NT Read Value.vi"("Name"="Target Distance") -> ("Numeric"=w521:dbl)  [unwired: 9 in, 1 out]
    n354 = call-poly <vilib>:"NT Write Value.vi"("Boolean"=w532, "Name"="Vision Toggle") -> ()  [unwired: 9 in, 1 out]
    n355 = Round To Nearest(number=w521) -> (nearest integer value=→"Target Distance":dbl)
    n356 = call-poly <vilib>:"NT Read Value.vi"("Default Value"=0.0, "Name"="Bottom RPM") -> ("Numeric"=w523:dbl)  [unwired: 8 in, 1 out]
    n357 = call-poly <vilib>:"NT Read Value.vi"("Name"="/limelight/ts") -> ("Numeric"=w515:dbl)  [unwired: 9 in, 1 out]
    n358 = call-poly <vilib>:"NT Read Value.vi"("Name"="/limelight/ta") -> ("Numeric"=w513:dbl)  [unwired: 9 in, 1 out]
    n359 = Round To Nearest(number=w523) -> (nearest integer value=→"Bottom RPM":dbl)
    n360 = Round To Nearest(number=w515) -> (nearest integer value=→"Skew":dbl)
    n361 = Round To Nearest(number=w513) -> (nearest integer value=→"Area":dbl)
  }
